vi "TEB Processed= Message.vi"(0 "Module Name":string, 1 "Event Number":i32) -> ()   [LabVIEW 2009]
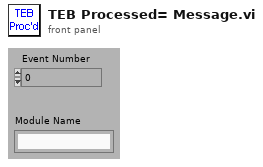
[diagram p1: front panel]
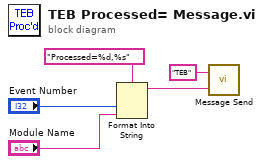
[diagram p0: block diagram]
diagram:
  n1 = Format Into String(format string="Processed=%d,%s" ("Format String"), "Event Number", "Module Name") -> (resulting string=w2:string)  [unwired: 2 in, 1 out]
  n2 = call "Message Send.vi"("Message"=w2, "Destination"="TEB") -> ()
